vi "AR-Interlock-parse.vi"(8 "error in":errorcluster, 10 "Perv uS time":u32, 11 "Str in":string="GI,79,1559115186,0,0,1,0,0,0\r\n\n") -> (0 "error out":errorcluster, 1 "Head R Edge":bool, 2 "Head F Edge":bool, 3 "Intlk Data":T1 {"Time Delta (mS)" format="%.3f"})   [LabVIEW 2021]
uses:
  Controls/AR-Interlock-Data.ctl
panel:
  # "GI,79,1559115186,0,0,1,0,0,0\nGI,80,1559697243,0,0,1,0,0,0\nGI,81,1574721570,1,1,1,0,0,0\nGI,82,1574986528,0,0,1,0,0,1\nGI,83,1593927425,1,1,1,0,0,0\nGI,84,1594078331,0,0,1,0,0,1\nGI,85,1595749995,1,1,1,0,0,0\nGI,86,1595923174,0,0,1,0,0,1"
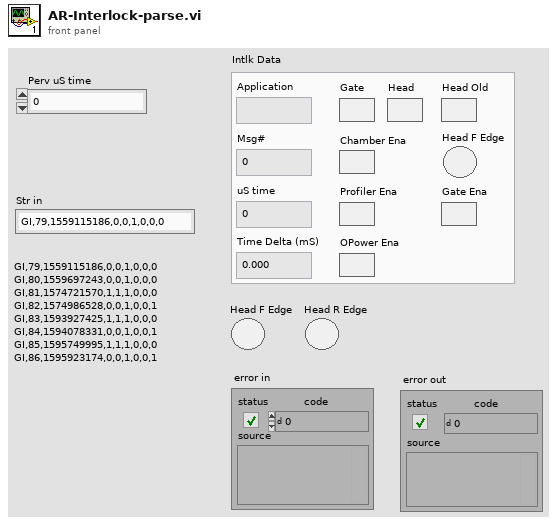
[diagram p1: front panel]
types:
  T1 = typedef "AR-Interlock-Data.ctl" = cluster{"Application":string, "Msg#":i32, "uS time":u32, "Gate":bool, "Head":bool, "Head Old":bool, "Chamber Ena":bool, "Profiler Ena":bool, "OPower Ena":bool, "Gate Ena":bool, "Time Delta (mS)":dbl, "Head F Edge":bool}
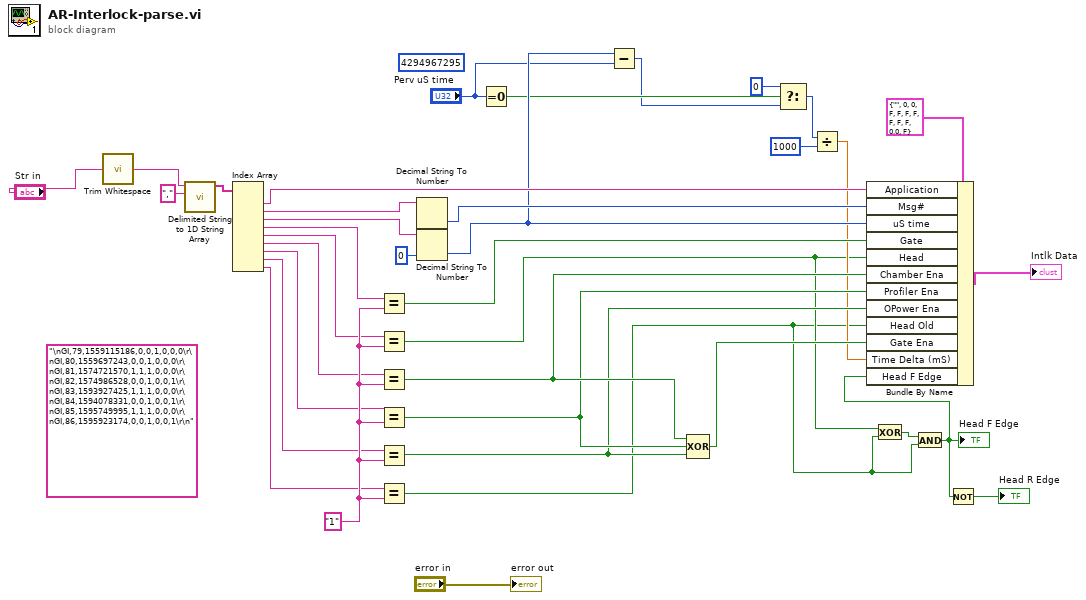
[diagram p0: block diagram]
diagram:
  (unwired) "\nGI,79,1559115186,0,0,1,0,0,0\r\nGI,80,1559697243,0,0,1,0,0,0\r\nGI,81,1574721570,1,1,1,0,0,0\r\nGI,82,1574986528,0,0,1,0,0,1\r\nGI,83,1593927425,1,1,1,0,0,0\r\nGI,84,1594078331,0,0,1,0,0,1\r\nGI,85,1595749995,1,1,1,0,0,0\r\nGI,86,1595923174,0,0,1,0,0,1\r\n" ("Output")
  (unwired) u32 4294967295
  w30 = "1"
  n1 = call <vilib>:"Trim Whitespace.vi"("string"="Str in") -> ("trimmed string"=w15:string)  [unwired: 1 in]
  n2 = call <vilib>:"Delimited String to 1D String Array.vi"("delimiter"=",", "delimited string"=w15) -> ("string array"=w36:string[])  [unwired: 9 in]
  n3 = Index Array(array=w36) -> (element #1=w35:string, element #2=w34:string, element #3=w32:string, element #4=w31:string, element #5=w29:string, element #6=w20:string, element #7=w19:string, element #8=w18:string, element #9=w17:string)  [unwired: 9 in]
  n4 = Equal?(x=w31, y=w30) -> (x = y?=w28:bool)
  n5 = Equal?(x=w29, y=w30) -> (x = y?=w5:bool)
  n6 = Equal?(x=w20, y=w30) -> (x = y?=w27:bool)
  n7 = Equal?(x=w19, y=w30) -> (x = y?=w26:bool)
  n8 = Equal?(x=w18, y=w30) -> (x = y?=w25:bool)
  n9 = Equal?(x=w17, y=w30) -> (x = y?=w4:bool)
  n10 = Decimal String To Number(string=w34) -> (number=w33:i32)  [unwired: 2 in, 1 out]
  n11 = Decimal String To Number(string=w32, default (0L)=u32 0 ("default (0 I32)")) -> (number=w23:u32)  [unwired: 1 in, 1 out]
  n12 = Equal To 0?(x="Perv uS time") -> (x = 0?=w22:bool)
  n13 = Subtract(x=w23, y="Perv uS time") -> (x-y=w10:u32)
  n14 = Compound Arithmetic op=XOR(w27, w26, w25) -> (w24:bool)
  n15 = Select(t=u32 0, s=w22, f=w10) -> (s? t:f=w14:u32)
  n16 = Divide(x=w14, y=u32 1000) -> (x/y=w12:dbl)
  n17 = Exclusive Or(1:w4, 2:w5) -> (0:w6:bool)
  n18 = And(x=w6, y=w4) -> (x .and. y?=w1:bool)
  "Head F Edge" <- w1
  n19 = Bundle By Name(cluster=T1 {"Application"="", "Msg#"=0, "uS time"=0, "Gate"=FALSE, "Head"=FALSE, "Head Old"=FALSE, "Chamber Ena"=FALSE, "Profiler Ena"=FALSE, "OPower Ena"=FALSE, "Gate Ena"=FALSE, "Time Delta (mS)"=0.0, "Head F Edge"=FALSE} ("Intlk Data"), "Application"=w35, "Msg#"=w33, "uS time"=w23, "Gate"=w28, "Head"=w5, "Chamber Ena"=w27, "Profiler Ena"=w26, "OPower Ena"=w25, "Head Old"=w4, "Gate Ena"=w24, "Time Delta (mS)"=w12, "Head F Edge"=w1) -> (→"Intlk Data":T1)
  n20 = Not(x=w1) -> (.not. x?=→"Head R Edge":bool)
  "error out" <- "error in"
